vi "Create IO Channels.vi"(6 "AI Buffer Size (s)":i32=10, 8 "AI Block Size":i32=5000, 9 "OSC Configuration":T3(array[cluster])=[[{"Signal Type"=enum."Sine Wave", "DC"=0.0, "Amplitude"=0.01, "frequency"=2.0, "Phase"=0.0}, {"Signal Type"=enum."Sine Wave", "DC"=0.001, "Amplitude"=0.005, "frequency"=2.0, "Phase"=0.0}]] {"frequency" step=0.001 format="%.3p"; "Amplitude" format="%0.2p"; "DC" min=-0.99 max=0.99 format="%.2p"}, 10 "AO Configuration":T1(array[cluster])=[{"Output physical channels"="PXI1Slot2/ao0", "AO. Max"=0.1, "AO.Min"=-0.1}, {"Output physical channels"="", "AO. Max"=0.1, "AO.Min"=-0.1}], 11 "AI Configuration":T2(array[cluster])=[{"AI.Coupling"=10050, "AI.Max"=10.0, "AI.Min"=-10.0, "Input physical channels"="PXI1Slot2/ai0:1"}, {"AI.Coupling"=10050, "AI.Max"=10.0, "AI.Min"=-10.0, "Input physical channels"="PXI1Slot3/ai0:3"}, {"AI.Coupling"=10050, "AI.Max"=10.0, "AI.Min"=-10.0, "Input physical channels"=""}] {"AI.Coupling" items=["AC"=10045, "DC"=10050, "GND"=10066]}) -> (0 "sampling info":cluster{"Fs":dbl, "#s":dbl}, 1 "AI Rate":dbl=10000.0 format="%.2f", 2 "AO Task":refnum<k21>[](array[refnum]), 3 "AI task":refnum<k21>[](array[refnum]), 4 "phase log":dbl[](array[numeric])=[0.99999999999938, 0.99999999999938], 5 "appended array":errorcluster[][](array[cluster]))   [LabVIEW 2013]
uses:
  <vilib>/DAQmx/configure/timing.llb/DAQmx Timing (Sample Clock).vi
  <vilib>/DAQmx/create/channels.llb/DAQmx Create Channel (AI-Voltage-Basic).vi
  <vilib>/DAQmx/write.llb/DAQmx Write (Analog 1D Wfm NChan NSamp).vi
  <resource>/objmgr/daqmx.rc
  <vilib>/DAQmx/configure/trigger.llb/DAQmx Start Trigger (Digital Edge).vi
  <vilib>/measure/NI_MABase.lvlib
  <vilib>/DAQmx/create/channels.llb/DAQmx Create Channel (AO-Voltage-Basic).vi
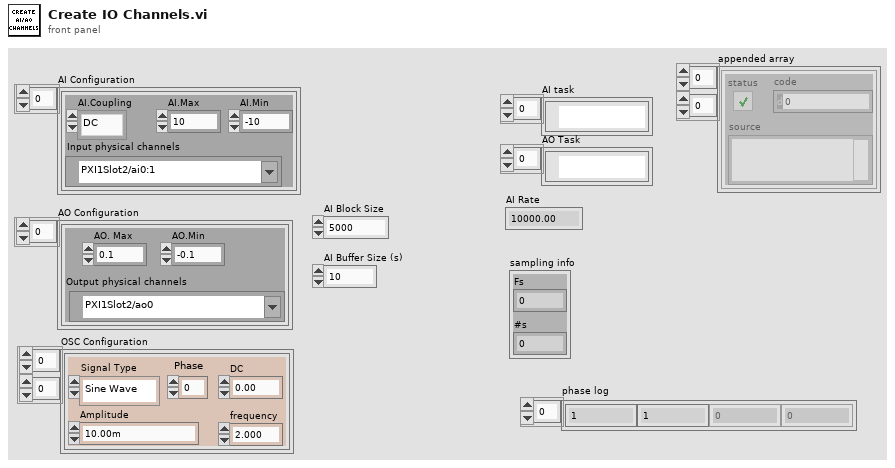
[diagram p1: front panel]
types:
  T1 = cluster{"Output physical channels":tag, "AO. Max":dbl, "AO.Min":dbl}[]
  T2 = cluster{"AI.Coupling":i32, "AI.Max":dbl, "AI.Min":dbl, "Input physical channels":tag}[]
  T3 = cluster{"Signal Type":enum16{"Sine Wave", "Triangle Wave", "Square Wave", "Sawtooth Wave"}, "DC":dbl, "Amplitude":dbl, "frequency":dbl, "Phase":dbl}[][]
  T4 = cluster{"Output physical channels":tag, "AO. Max":dbl, "AO.Min":dbl}
  T5 = cluster{"AI.Coupling":i32, "AI.Max":dbl, "AI.Min":dbl, "Input physical channels":tag}
  T6 = cluster{"Signal Type":enum16{"Sine Wave", "Triangle Wave", "Square Wave", "Sawtooth Wave"}, "DC":dbl, "Amplitude":dbl, "frequency":dbl, "Phase":dbl}
  T7 = enum16{"Sine Wave", "Triangle Wave", "Square Wave", "Sawtooth Wave"}
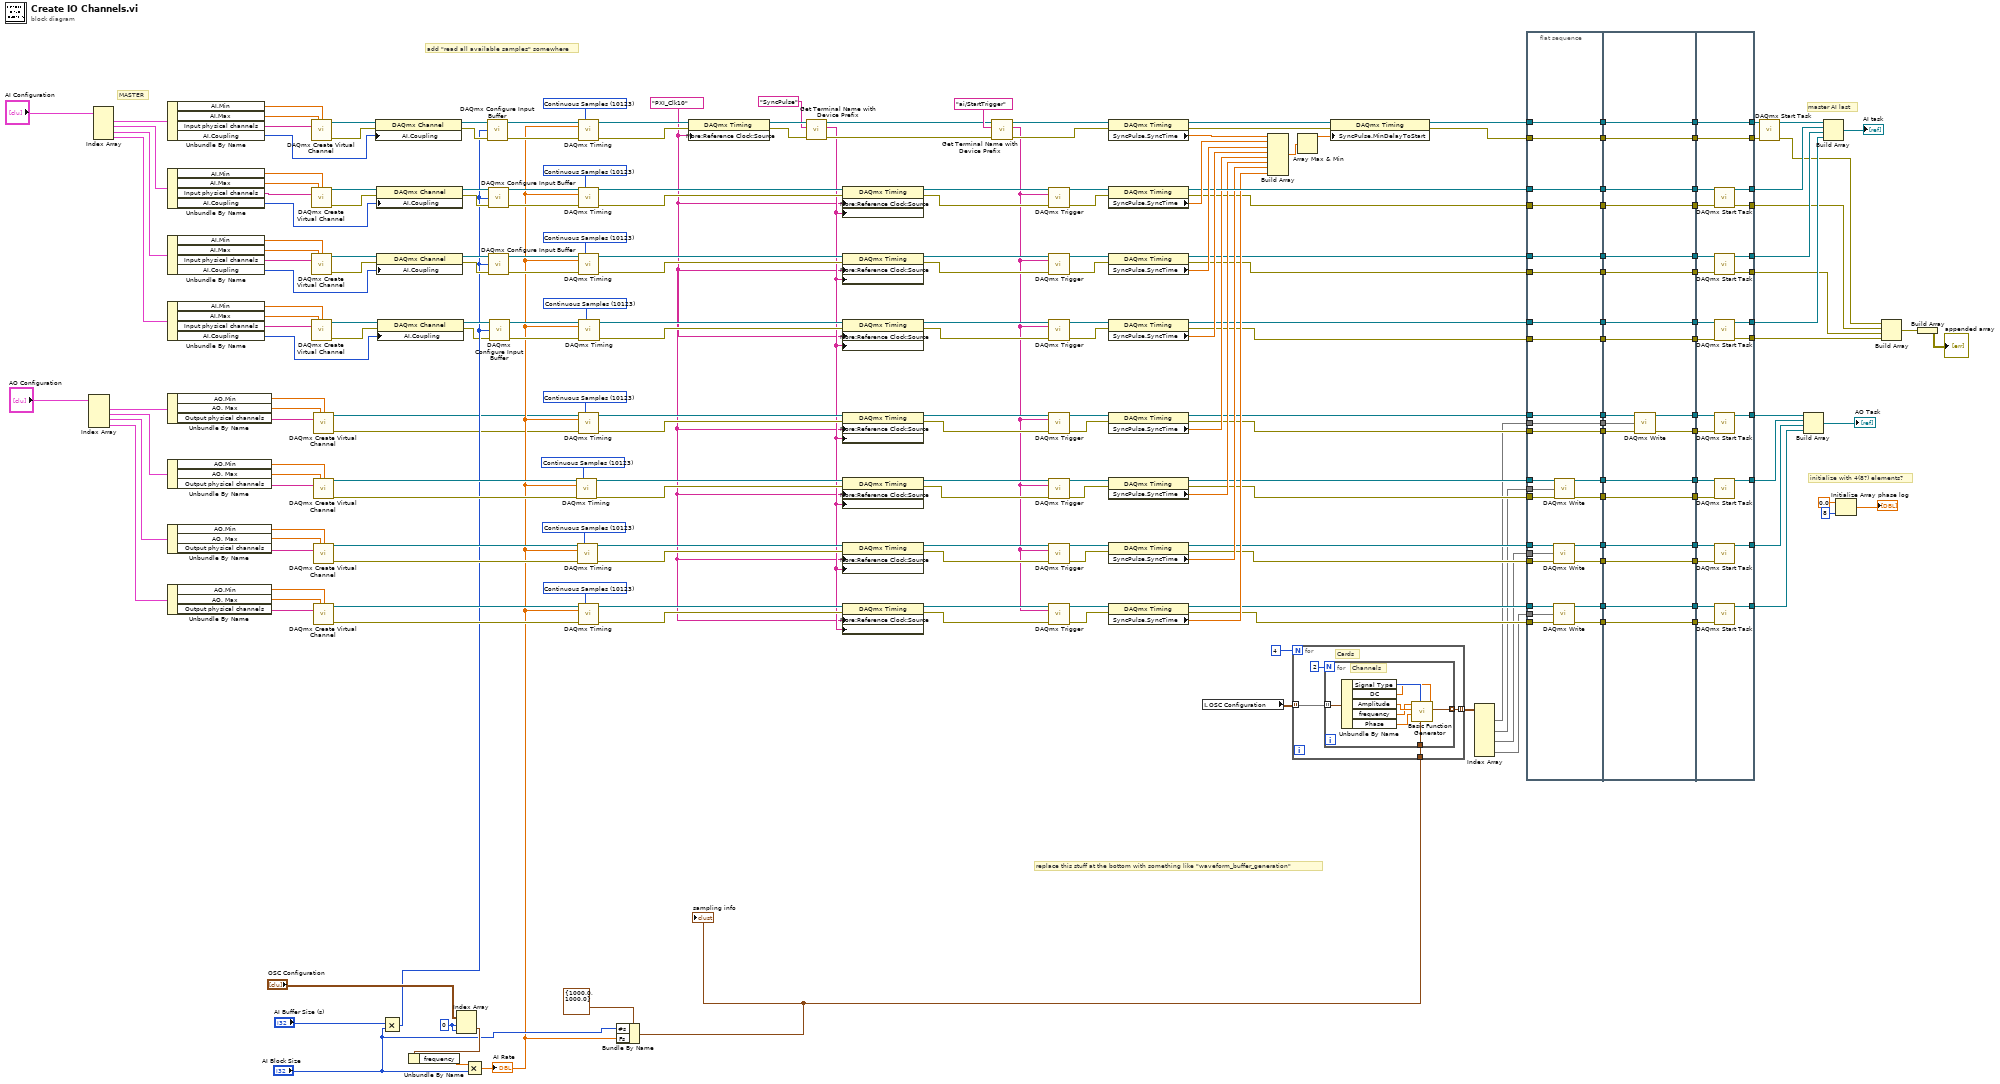
[diagram p0: block diagram]
diagram:
  w5 = tag "PXI_Clk10" ("RefClk.Src")
  w87 = 10123 items=["Finite Samples"=10178, "Continuous Samples"=10123] ("sample mode")
  w102 = 10123 items=["Finite Samples"=10178, "Continuous Samples"=10123] ("sample mode")
  w111 = 10123 items=["Finite Samples"=10178, "Continuous Samples"=10123] ("sample mode")
  w125 = 10123 items=["Finite Samples"=10178, "Continuous Samples"=10123] ("sample mode")
  w152 = 10123 items=["Finite Samples"=10178, "Continuous Samples"=10123] ("sample mode")
  w168 = 10123 items=["Finite Samples"=10178, "Continuous Samples"=10123] ("sample mode")
  w181 = 10123 items=["Finite Samples"=10178, "Continuous Samples"=10123] ("sample mode")
  w198 = 0 ("index (row)")
  w227 = 10123 items=["Finite Samples"=10178, "Continuous Samples"=10123] ("sample mode")
  # "master AI last"
  # "replace this stuff at the bottom with something like \"waveform_buffer_generation\""
  # "initialize with 4(8?) elements?"
  # "add \"read all available samples\" somewhere"
  # "MASTER"
  n1 = Index Array(array="AO Configuration") -> (element #1=w129:T4, element #2=w80:T4, element #3=w81:T4, element #4=w82:T4)  [unwired: 4 in]
  n2 = Index Array(array="AI Configuration") -> (element #1=w228:T5, element #2=w182:T5, element #3=w145:T5, element #4=w144:T5)  [unwired: 4 in]
  n3 = Unbundle By Name(w228) -> ("AI.Min"=w193:dbl, "AI.Max"=w194:dbl, "Input physical channels"=w212:tag, "AI.Coupling"=w192:i32)
  n4 = Unbundle By Name(w182) -> ("AI.Min"=w189:dbl, "AI.Max"=w188:dbl, "Input physical channels"=w183:tag, "AI.Coupling"=w190:i32)
  n5 = Unbundle By Name(w145) -> ("AI.Min"=w161:dbl, "AI.Max"=w162:dbl, "Input physical channels"=w167:tag, "AI.Coupling"=w160:i32)
  n6 = Unbundle By Name(w144) -> ("AI.Min"=w158:dbl, "AI.Max"=w157:dbl, "Input physical channels"=w153:tag, "AI.Coupling"=w159:i32)
  n7 = Unbundle By Name(w129) -> ("AO.Min"=w126:dbl, "AO. Max"=w127:dbl, "Output physical channels"=w128:tag)
  n8 = Unbundle By Name(w80) -> ("AO.Min"=w109:dbl, "AO. Max"=w108:dbl, "Output physical channels"=w107:tag)
  n9 = Unbundle By Name(w81) -> ("AO.Min"=w104:dbl, "AO. Max"=w105:dbl, "Output physical channels"=w106:tag)
  n10 = Unbundle By Name(w82) -> ("AO.Min"=w85:dbl, "AO. Max"=w84:dbl, "Output physical channels"=w83:tag)
  n11 = call-poly <vilib>:"DAQmx Create Virtual Channel.vi"("maximum value"=w194, "minimum value"=w193, "physical channels"=w212) -> ("task out"=w211:refnum<k21>, "error out"=w210:errorcluster)  [unwired: 11 in]
  n12 = call-poly <vilib>:"DAQmx Create Virtual Channel.vi"("maximum value"=w188, "minimum value"=w189, "physical channels"=w183) -> ("task out"=w184:refnum<k21>, "error out"=w185:errorcluster)  [unwired: 11 in]
  n13 = call-poly <vilib>:"DAQmx Create Virtual Channel.vi"("maximum value"=w162, "minimum value"=w161, "physical channels"=w167) -> ("task out"=w166:refnum<k21>, "error out"=w165:errorcluster)  [unwired: 11 in]
  n14 = call-poly <vilib>:"DAQmx Create Virtual Channel.vi"("maximum value"=w157, "minimum value"=w158, "physical channels"=w153) -> ("task out"=w154:refnum<k21>, "error out"=w155:errorcluster)  [unwired: 11 in]
  n15 = call-poly <vilib>:"DAQmx Create Virtual Channel.vi"("maximum value"=w127, "minimum value"=w126, "physical channels"=w128) -> ("task out"=w3:refnum<k21>, "error out"=w1:errorcluster)  [unwired: 11 in]
  n16 = call-poly <vilib>:"DAQmx Create Virtual Channel.vi"("maximum value"=w108, "minimum value"=w109, "physical channels"=w107) -> ("task out"=w110:refnum<k21>, "error out"=w112:errorcluster)  [unwired: 11 in]
  n17 = call-poly <vilib>:"DAQmx Create Virtual Channel.vi"("maximum value"=w105, "minimum value"=w104, "physical channels"=w106) -> ("task out"=w103:refnum<k21>, "error out"=w101:errorcluster)  [unwired: 11 in]
  n18 = call-poly <vilib>:"DAQmx Create Virtual Channel.vi"("maximum value"=w84, "minimum value"=w85, "physical channels"=w83) -> ("task out"=w86:refnum<k21>, "error out"=w88:errorcluster)  [unwired: 11 in]
  n19 = property class="DAQmx Channel"(reference=w211, error in=w210, "AI.Coupling"=w192) -> (reference out=w209:refnum<k21>, error out=w208:errorcluster)
  n20 = property class="DAQmx Channel"(reference=w184, error in=w185, "AI.Coupling"=w190) -> (reference out=w186:refnum<k21>, error out=w187:errorcluster)
  n21 = property class="DAQmx Channel"(reference=w166, error in=w165, "AI.Coupling"=w160) -> (reference out=w164:refnum<k21>, error out=w163:errorcluster)
  n22 = property class="DAQmx Channel"(reference=w154, error in=w155, "AI.Coupling"=w159) -> (reference out=w156:refnum<k21>, error out=w10:errorcluster)
  n23 = Multiply(x="AI Buffer Size (s)", y="AI Block Size") -> (x*y=w11:i32)
  n24 = Index Array(array="OSC Configuration", index (row)=w198, index (col)=w198) -> (element=w202:T6)
  n25 = Unbundle By Name(w202) -> ("frequency"=w201:dbl)
  n26 = Multiply(x=w201, y="AI Block Size") -> (x*y=w75:dbl)
  "AI Rate" <- w75
  n27 = call <vilib>:"DAQmx Configure Input Buffer.vi"("task/channels in"=w209, "buffer size (in samples per channel)"=w11, "error in"=w208) -> ("task out"=w207:refnum<k21>, "error out"=w206:errorcluster)  [unwired: 11 in]
  n28 = call <vilib>:"DAQmx Configure Input Buffer.vi"("task/channels in"=w186, "buffer size (in samples per channel)"=w11, "error in"=w187) -> ("task out"=w180:refnum<k21>, "error out"=w179:errorcluster)  [unwired: 11 in]
  n29 = call <vilib>:"DAQmx Configure Input Buffer.vi"("task/channels in"=w164, "buffer size (in samples per channel)"=w11, "error in"=w163) -> ("task out"=w169:refnum<k21>, "error out"=w170:errorcluster)  [unwired: 11 in]
  n30 = call <vilib>:"DAQmx Configure Input Buffer.vi"("task/channels in"=w156, "buffer size (in samples per channel)"=w11, "error in"=w10) -> ("task out"=w151:refnum<k21>, "error out"=w150:errorcluster)  [unwired: 11 in]
  n31 = call-poly <vilib>:"DAQmx Timing.vi"("task/channels in"=w110, "sample mode"=w111, "rate"=w75, "error in"=w112) -> ("task out"=w114:refnum<k21>, "error out"=w115:errorcluster)  [unwired: 10 in]
  n32 = call-poly <vilib>:"DAQmx Timing.vi"("task/channels in"=w103, "sample mode"=w102, "rate"=w75, "error in"=w101) -> ("task out"=w99:refnum<k21>, "error out"=w98:errorcluster)  [unwired: 10 in]
  n33 = call-poly <vilib>:"DAQmx Timing.vi"("task/channels in"=w207, "sample mode"=w227, "rate"=w75, "error in"=w206) -> ("task out"=w226:refnum<k21>, "error out"=w191:errorcluster)  [unwired: 10 in]
  n34 = call-poly <vilib>:"DAQmx Timing.vi"("task/channels in"=w180, "sample mode"=w181, "rate"=w75, "error in"=w179) -> ("task out"=w178:refnum<k21>, "error out"=w177:errorcluster)  [unwired: 10 in]
  n35 = call-poly <vilib>:"DAQmx Timing.vi"("task/channels in"=w169, "sample mode"=w168, "rate"=w75, "error in"=w170) -> ("task out"=w171:refnum<k21>, "error out"=w172:errorcluster)  [unwired: 10 in]
  n36 = call-poly <vilib>:"DAQmx Timing.vi"("task/channels in"=w3, "sample mode"=w125, "rate"=w75, "error in"=w1) -> ("task out"=w123:refnum<k21>, "error out"=w122:errorcluster)  [unwired: 10 in]
  n37 = call-poly <vilib>:"DAQmx Timing.vi"("task/channels in"=w86, "sample mode"=w87, "rate"=w75, "error in"=w88) -> ("task out"=w90:refnum<k21>, "error out"=w91:errorcluster)  [unwired: 10 in]
  n38 = call-poly <vilib>:"DAQmx Timing.vi"("task/channels in"=w151, "sample mode"=w152, "rate"=w75, "error in"=w150) -> ("task out"=w149:refnum<k21>, "error out"=w148:errorcluster)  [unwired: 10 in]
  n39 = Bundle By Name(cluster=cluster{"Fs":dbl, "#s":dbl} {"Fs"=1000.0, "#s"=1000.0} ("sampling info"), "#s"="AI Block Size", "Fs"=w75) -> (w2:cluster{"Fs":dbl, "#s":dbl})
  "sampling info" <- w2
  n40 = property class="DAQmx Timing"(reference=w226, error in=w191, "More:Reference Clock:Source"=w5) -> (reference out=w9:refnum<k21>, error out=w8:errorcluster)
  n41 = call "Get Terminal Name with Device Prefix.vi"("error in (no error)"=w8, "Local Terminal Name"="SyncPulse", "task/channels in"=w9) -> ("error out"=w221:errorcluster, "Terminal Name with Device Prefix"=w6:tag, "task out"=w222:refnum<k21>)  [unwired: 6 in]
  n42 = property class="DAQmx Timing"(reference=w178, error in=w177, "More:Reference Clock:Source"=w5, "More:Synchronization Pulse:Source"=w6) -> (reference out=w176:refnum<k21>, error out=w175:errorcluster)
  n43 = property class="DAQmx Timing"(reference=w171, error in=w172, "More:Reference Clock:Source"=w5, "More:Synchronization Pulse:Source"=w6) -> (reference out=w173:refnum<k21>, error out=w174:errorcluster)
  n44 = property class="DAQmx Timing"(reference=w149, error in=w148, "More:Reference Clock:Source"=w5, "More:Synchronization Pulse:Source"=w6) -> (reference out=w147:refnum<k21>, error out=w146:errorcluster)
  n45 = property class="DAQmx Timing"(reference=w123, error in=w122, "More:Reference Clock:Source"=w5, "More:Synchronization Pulse:Source"=w6) -> (reference out=w124:refnum<k21>, error out=w121:errorcluster)
  n46 = property class="DAQmx Timing"(reference=w114, error in=w115, "More:Reference Clock:Source"=w5, "More:Synchronization Pulse:Source"=w6) -> (reference out=w113:refnum<k21>, error out=w116:errorcluster)
  n47 = property class="DAQmx Timing"(reference=w99, error in=w98, "More:Reference Clock:Source"=w5, "More:Synchronization Pulse:Source"=w6) -> (reference out=w100:refnum<k21>, error out=w97:errorcluster)
  n48 = property class="DAQmx Timing"(reference=w90, error in=w91, "More:Reference Clock:Source"=w5, "More:Synchronization Pulse:Source"=w6) -> (reference out=w89:refnum<k21>, error out=w92:errorcluster)
  n49 = call "Get Terminal Name with Device Prefix.vi"("error in (no error)"=w221, "Local Terminal Name"="ai/StartTrigger", "task/channels in"=w222) -> ("error out"=w219:errorcluster, "Terminal Name with Device Prefix"=w74:tag, "task out"=w220:refnum<k21>)  [unwired: 6 in]
  n50 = call-poly <vilib>:"DAQmx Trigger.vi"("task/channels in"=w176, "source"=w74, "error in"=w175) -> ("task out"=w141:refnum<k21>, "error out"=w140:errorcluster)  [unwired: 11 in]
  n51 = call-poly <vilib>:"DAQmx Trigger.vi"("task/channels in"=w173, "source"=w74, "error in"=w174) -> ("task out"=w142:refnum<k21>, "error out"=w139:errorcluster)  [unwired: 11 in]
  n52 = call-poly <vilib>:"DAQmx Trigger.vi"("task/channels in"=w147, "source"=w74, "error in"=w146) -> ("task out"=w143:refnum<k21>, "error out"=w138:errorcluster)  [unwired: 11 in]
  n53 = call-poly <vilib>:"DAQmx Trigger.vi"("task/channels in"=w124, "source"=w74, "error in"=w121) -> ("task out"=w120:refnum<k21>, "error out"=w119:errorcluster)  [unwired: 11 in]
  n54 = call-poly <vilib>:"DAQmx Trigger.vi"("task/channels in"=w113, "source"=w74, "error in"=w116) -> ("task out"=w117:refnum<k21>, "error out"=w118:errorcluster)  [unwired: 11 in]
  n55 = call-poly <vilib>:"DAQmx Trigger.vi"("task/channels in"=w100, "source"=w74, "error in"=w97) -> ("task out"=w96:refnum<k21>, "error out"=w95:errorcluster)  [unwired: 11 in]
  n56 = call-poly <vilib>:"DAQmx Trigger.vi"("task/channels in"=w89, "source"=w74, "error in"=w92) -> ("task out"=w93:refnum<k21>, "error out"=w94:errorcluster)  [unwired: 11 in]
  n57 = property class="DAQmx Timing"(reference=w220, error in=w219) -> (reference out=w216:refnum<k21>, error out=w217:errorcluster, "SyncPulse.SyncTime"=w218:dbl)
  n58 = property class="DAQmx Timing"(reference=w141, error in=w140) -> (reference out=w131:refnum<k21>, error out=w65:errorcluster, "SyncPulse.SyncTime"=w136:dbl)
  n59 = property class="DAQmx Timing"(reference=w142, error in=w139) -> (reference out=w71:refnum<k21>, error out=w62:errorcluster, "SyncPulse.SyncTime"=w135:dbl)
  n60 = property class="DAQmx Timing"(reference=w143, error in=w138) -> (reference out=w68:refnum<k21>, error out=w59:errorcluster, "SyncPulse.SyncTime"=w134:dbl)
  n61 = property class="DAQmx Timing"(reference=w120, error in=w119) -> (reference out=w56:refnum<k21>, error out=w47:errorcluster, "SyncPulse.SyncTime"=w79:dbl)
  n62 = property class="DAQmx Timing"(reference=w117, error in=w118) -> (reference out=w53:refnum<k21>, error out=w45:errorcluster, "SyncPulse.SyncTime"=w78:dbl)
  n63 = property class="DAQmx Timing"(reference=w96, error in=w95) -> (reference out=w50:refnum<k21>, error out=w42:errorcluster, "SyncPulse.SyncTime"=w77:dbl)
  n64 = property class="DAQmx Timing"(reference=w93, error in=w94) -> (reference out=w39:refnum<k21>, error out=w36:errorcluster, "SyncPulse.SyncTime"=w76:dbl)
  n65 = local read "OSC Configuration"() -> (w199:T3)
  n66 = Build Array(w218, w136, w135, w134, w79, w78, w77, w76) -> (w215:dbl[])
  n67 = for {
    N: 4 -> [_]
    tunnel: w199 -> [w236] mode=indexing
    tunnel: [w235] -> w26 mode=indexing
    tunnel: w2 -> [w233]
    # "Cards"
    n68 = for {
      N: 2 -> [_]
      tunnel: w236 -> [w238] mode=indexing
      tunnel: [w239] -> w235 mode=indexing
      tunnel: w233 -> [w237]
      # "Channels"
      n69 = Unbundle By Name(w238) -> ("Signal Type"=w244:T7, "DC"=w243:dbl, "Amplitude"=w242:dbl, "frequency"=w241:dbl, "Phase"=w240:dbl)
      n70 = call <vilib>:"Basic Function Generator.vi"("offset"=w243, "sampling info"=w237, "signal type"=w244, "phase"=w240, "amplitude"=w242, "frequency"=w241) -> ("signal out"=w239:waveform(dbl))  [unwired: 3 in, 2 out]
    }
  }
  n71 = Array Max & Min(array=w215) -> (max value=w137:dbl)  [unwired: 3 out]
  n72 = property class="DAQmx Timing"(reference=w216, error in=w217, "SyncPulse.MinDelayToStart"=w137) -> (reference out=w213:refnum<k21>, error out=w214:errorcluster)
  n73 = Index Array(array=w26) -> (element #1=w24:waveform(dbl)[], element #2=w23:waveform(dbl)[], element #3=w22:waveform(dbl)[], element #4=w21:waveform(dbl)[])  [unwired: 8 in]
  n74 = flat-sequence {
    tunnel: w214 -> [w269]
    tunnel: w213 -> [w270]
    tunnel: [w270] -> w232
    tunnel: [w269] -> w231
    tunnel: [w268] -> w132
    tunnel: w131 -> [w268]
    tunnel: [w267] -> w72
    tunnel: w71 -> [w267]
    tunnel: [w266] -> w69
    tunnel: w68 -> [w266]
    tunnel: [w265] -> w66
    tunnel: w65 -> [w265]
    tunnel: [w264] -> w63
    tunnel: w62 -> [w264]
    tunnel: [w263] -> w60
    tunnel: w59 -> [w263]
    tunnel: [w262] -> w57
    tunnel: w56 -> [w262]
    tunnel: [w250] -> w54
    tunnel: w53 -> [w251]
    tunnel: [w254] -> w51
    tunnel: w50 -> [w253]
    tunnel: [w261] -> w48
    tunnel: w47 -> [w261]
    tunnel: w45 -> [w252]
    tunnel: [w255] -> w43
    tunnel: w42 -> [w256]
    tunnel: [w257] -> w40
    tunnel: w39 -> [w260]
    tunnel: [w258] -> w37
    tunnel: w36 -> [w259]
    tunnel: [w249] -> w35
    tunnel: [w248] -> w25
    tunnel: w24 -> [w248]
    tunnel: w23 -> [w247]
    tunnel: w22 -> [w246]
    tunnel: w21 -> [w245]
    tunnel: [w289] -> w230
    tunnel: [w288] -> w229
    tunnel: w232 -> [w289]
    tunnel: w231 -> [w288]
    tunnel: [w287] -> w133
    tunnel: w132 -> [w287]
    tunnel: [w286] -> w73
    tunnel: w72 -> [w286]
    tunnel: [w285] -> w70
    tunnel: w69 -> [w285]
    tunnel: [w284] -> w67
    tunnel: w66 -> [w284]
    tunnel: [w283] -> w64
    tunnel: w63 -> [w283]
    tunnel: [w282] -> w61
    tunnel: w60 -> [w282]
    tunnel: [w274] -> w58
    tunnel: w57 -> [w275]
    tunnel: [w281] -> w55
    tunnel: w54 -> [w281]
    tunnel: [w280] -> w52
    tunnel: w51 -> [w280]
    tunnel: [w273] -> w49
    tunnel: w48 -> [w272]
    tunnel: [w279] -> w46
    tunnel: [w278] -> w44
    tunnel: w43 -> [w278]
    tunnel: [w277] -> w41
    tunnel: w40 -> [w277]
    tunnel: [w276] -> w38
    tunnel: w37 -> [w276]
    tunnel: w35 -> [w279]
    tunnel: w25 -> [w271]
    tunnel: [w315] -> w225
    tunnel: [w314] -> w224
    tunnel: w230 -> [w315]
    tunnel: w229 -> [w314]
    tunnel: w133 -> [w313]
    tunnel: w73 -> [w312]
    tunnel: w70 -> [w311]
    tunnel: w67 -> [w310]
    tunnel: w64 -> [w309]
    tunnel: w61 -> [w308]
    tunnel: w58 -> [w307]
    tunnel: w55 -> [w306]
    tunnel: w52 -> [w305]
    tunnel: w49 -> [w304]
    tunnel: w46 -> [w303]
    tunnel: w44 -> [w302]
    tunnel: w41 -> [w301]
    tunnel: w38 -> [w300]
    tunnel: [w299] -> w34
    tunnel: [w298] -> w33
    tunnel: [w297] -> w32
    tunnel: [w296] -> w31
    tunnel: [w295] -> w30
    tunnel: [w294] -> w29
    tunnel: [w293] -> w28
    tunnel: [w292] -> w19
    tunnel: [w291] -> w16
    tunnel: [w290] -> w18
    frame #0 {
      n75 = call-poly <vilib>:"DAQmx Write.vi"("task/channels in"=w253, "data"=w246, "error in"=w256) -> ("task out"=w254:refnum<k21>, "error out"=w255:errorcluster)  [unwired: 10 in, 1 out]
      n76 = call-poly <vilib>:"DAQmx Write.vi"("task/channels in"=w260, "data"=w245, "error in"=w259) -> ("task out"=w257:refnum<k21>, "error out"=w258:errorcluster)  [unwired: 10 in, 1 out]
      n77 = call-poly <vilib>:"DAQmx Write.vi"("task/channels in"=w251, "data"=w247, "error in"=w252) -> ("task out"=w250:refnum<k21>, "error out"=w249:errorcluster)  [unwired: 10 in, 1 out]
    }
    frame #1 {
      n78 = call-poly <vilib>:"DAQmx Write.vi"("task/channels in"=w275, "data"=w271, "error in"=w272) -> ("task out"=w274:refnum<k21>, "error out"=w273:errorcluster)  [unwired: 10 in, 1 out]
    }
    frame #2 {
      n79 = call <vilib>:"DAQmx Start Task.vi"("task/channels in"=w313, "error in"=w310) -> ("task out"=w299:refnum<k21>, "error out"=w292:errorcluster)  [unwired: 12 in]
      n80 = call <vilib>:"DAQmx Start Task.vi"("task/channels in"=w312, "error in"=w309) -> ("task out"=w298:refnum<k21>, "error out"=w291:errorcluster)  [unwired: 12 in]
      n81 = call <vilib>:"DAQmx Start Task.vi"("task/channels in"=w311, "error in"=w308) -> ("task out"=w297:refnum<k21>, "error out"=w290:errorcluster)  [unwired: 12 in]
      n82 = call <vilib>:"DAQmx Start Task.vi"("task/channels in"=w307, "error in"=w304) -> ("task out"=w296:refnum<k21>)  [unwired: 12 in, 1 out]
      n83 = call <vilib>:"DAQmx Start Task.vi"("task/channels in"=w306, "error in"=w303) -> ("task out"=w295:refnum<k21>)  [unwired: 12 in, 1 out]
      n84 = call <vilib>:"DAQmx Start Task.vi"("task/channels in"=w305, "error in"=w302) -> ("task out"=w294:refnum<k21>)  [unwired: 12 in, 1 out]
      n85 = call <vilib>:"DAQmx Start Task.vi"("task/channels in"=w301, "error in"=w300) -> ("task out"=w293:refnum<k21>)  [unwired: 12 in, 1 out]
    }
  }
  n86 = call <vilib>:"DAQmx Start Task.vi"("task/channels in"=w225, "error in"=w224) -> ("task out"=w204:refnum<k21>, "error out"=w4:errorcluster)  [unwired: 12 in]
  n87 = Build Array(w31, w30, w29, w28) -> (→"AO Task":refnum<k21>[])
  n88 = Build Array(w204, w34, w33, w32) -> (→"AI task":refnum<k21>[])
  n89 = Initialize Array(0.0 ("element"), 8 ("dimension size")) -> (→"phase log":dbl[])
  n90 = Build Array(w4, w19, w16, w18) -> (w17:errorcluster[])
  n91 = Build Array(w17) -> (→"appended array":errorcluster[][])
